vi "Select APUs.vi"(11 "IP":refnum<class "Engine Simulation IP.lvclass">[](array[class])) -> (3 "APUs":refnum<class "APU.lvclass">[](array[class]))   [LabVIEW 2013, in "APU.lvclass"]
uses:
  APU.lvclass
  Engine Simulation IP.lvclass
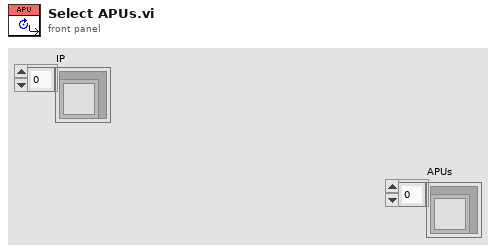
[diagram p1: front panel]
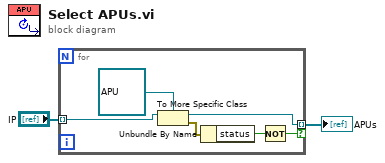
[diagram p0: block diagram]
diagram:
  n1 = for {
    tunnel: "IP" -> [w8] mode=indexing
    tunnel: [w3] -> w2 mode=indexing if=w4
    n2 = To More Specific Class(target class=refnum<class "APU.lvclass"> refnum ("APU.lvclass"), reference=w8) -> (specific class reference=w3:refnum<class "APU.lvclass">, error out=w6:errorcluster)  [unwired: 1 in]
    n3 = Unbundle By Name(w6) -> ("status"=w5:bool)
    n4 = Not(x=w5) -> (.not. x?=w4:bool)
  }
  "APUs" <- w2
